vi "get controller information.vi"(6 "Network Adapters (F)":bool caption="network adapters (F)", 8 "error in":errorcluster, 11 "controller in":refnum<class "Controller.lvclass">) -> (0 "error out":errorcluster, 2 "controller information":T1={"system session"=refnum, "system hardware ref"=refnum, "vendor name"="", "product name"="", "product ID"=0, "serial number"="", "device information"={"resource"="", "device class"="", "system start time"=timestamp(0 s since 1904-01-01), "current time"=timestamp(0 s since 1904-01-01), "time zone"="", "firmware revision"="", "image title"="", "image version"="", "system status"=""}, "primary network adapter"={"IP address"="", "MAC address"="", "IP address request mode"=1, "subnet mask"="", "gateway"="", "DNS server"="", "adapter mode"=1, "adapter type"=1}, "secondary network adapters"=[]} {"product ID" format="%.0x"; "primary network adapter"."IP address request mode" items=["Static"=1, "DHCP/Link Local"=2, "Link-Local Only"=4, "DHCP Only"=8]; "primary network adapter"."adapter type" items=["Ethernet"=1, "WLAN"=2]; "primary network adapter"."adapter mode" items=["Disabled"=1, "TCP/IP Ethernet"=2, "Deterministic"=4, "EtherCAT"=8, "TCP/IP WLAN Connect"=32, "TCP/IP WLAN Create"=64]; "secondary network adapters"."IP address request mode" items=["Static"=1, "DHCP/Link Local"=2, "Link-Local Only"=4, "DHCP Only"=8]; "secondary network adapters"."adapter type" items=["Disabled"=1, "TCP/IP Ethernet"=2, "Deterministic"=4, "EtherCAT"=8, "TCP/IP WLAN Connect"=32, "TCP/IP WLAN Create"=64]; "secondary network adapters"."adapter mode" items=["Disabled"=1, "TCP/IP Ethernet"=2, "Deterministic"=4, "EtherCAT"=8, "TCP/IP WLAN Connect"=32, "TCP/IP WLAN Create"=64]}, 3 "controller out":refnum<class "Controller.lvclass">)   [LabVIEW 2013, in "SMI.lvlib" / "Controller.lvclass"]
uses:
  Controller.lvclass
  controller information.ctl
  device information.ctl
  network adapter settings.ctl
  Controller.lvclass/Controller.ctl
  SysCfg Device/read system session.vi
  Device/read vendor name.vi
  Device/read product name.vi
  Device/read product ID.vi
  Device/read serial number.vi
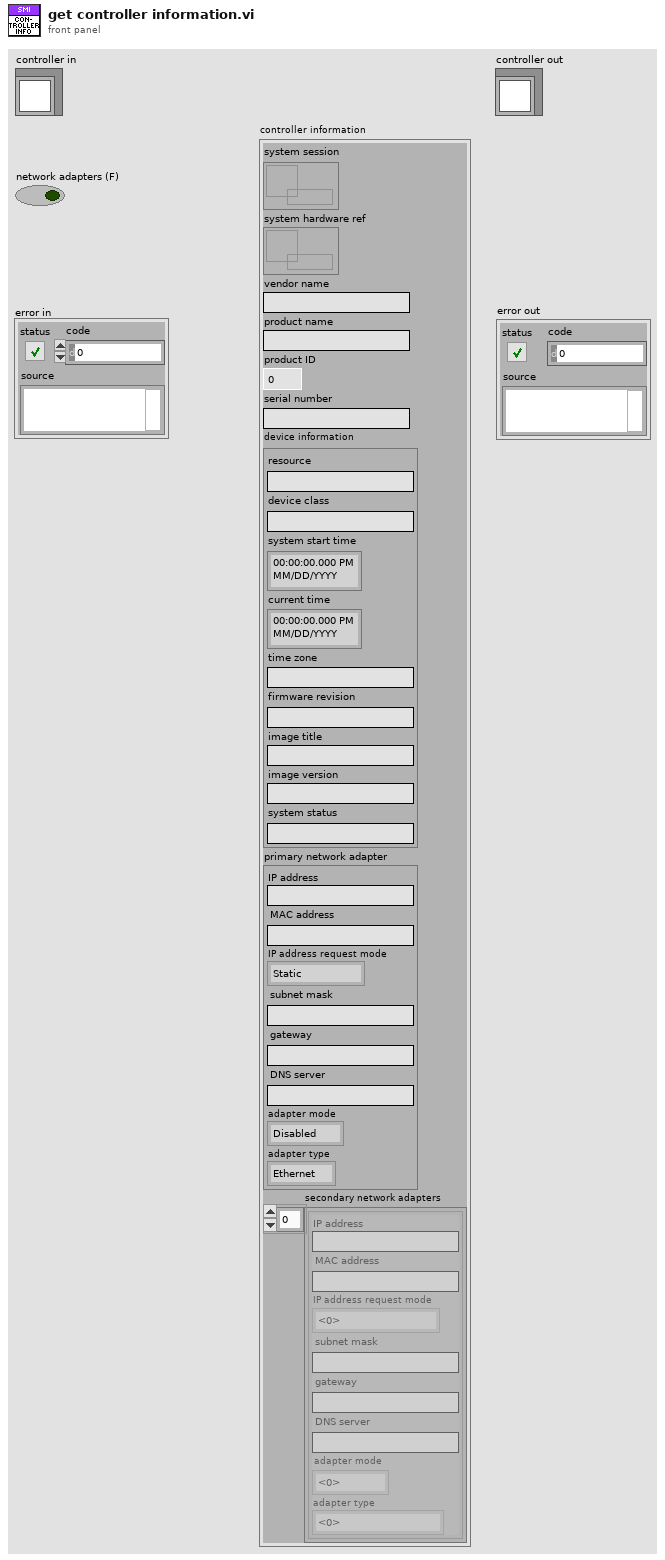
[diagram p1: front panel]
types:
  T1 = typedef "SMI.lvlib/Controller.lvclass/controller information.ctl" = cluster{"system session":refnum<data-value>, "system hardware ref":refnum<data-value>, "vendor name":string, "product name":string, "product ID":u16, "serial number":string, "device information":T2, "primary network adapter":T3, "secondary network adapters":T3[]}
  T2 = typedef "SMI.lvlib/Controller.lvclass/device information.ctl" = cluster{"resource":string, "device class":string, "system start time":timestamp, "current time":timestamp, "time zone":string, "firmware revision":string, "image title":string, "image version":string, "system status":string}
  T3 = typedef "SMI.lvlib/Controller.lvclass/network adapter settings.ctl" = cluster{"IP address":string, "MAC address":string, "IP address request mode":u32, "subnet mask":string, "gateway":string, "DNS server":string, "adapter mode":u32, "adapter type":u32}
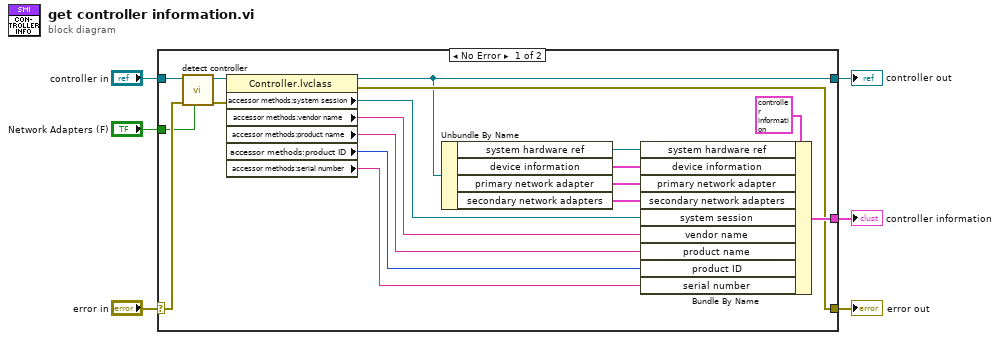
[diagram p0: block diagram]
diagram:
  n1 = case shown="No Error" "error in" {
    selector: "error in" -> [w11 w26]
    tunnel: [w24 _] -> w6
    tunnel: [w23 w26] -> w5
    tunnel: "controller in" -> [w8 w25]
    tunnel: [w13 w25] -> w4
    tunnel: "Network Adapters (F)" -> [w7 _]
    frame No Error {
      n2 = call "detect controller.vi"("Network Adapters"=w7, "error in"=w11, "controller in"=w8) -> ("error out"=w10:errorcluster, "controller out"=w9:refnum<class "Controller.lvclass">)  [unwired: 7 in]
      n3 = property class="Controller.lvclass"(reference=w9, error in=w10) -> (reference out=w13:refnum<class "Controller.lvclass">, error out=w23:errorcluster, "accessor methods:system session"=w12:refnum<data-value>, "accessor methods:vendor name"=w19:string, "accessor methods:product name"=w22:string, "accessor methods:product ID"=w21:u16, "accessor methods:serial number"=w20:string)
      n4 = Unbundle By Name(w13) -> ("system hardware ref"=w15:refnum<data-value>, "device information"=w18:T2, "primary network adapter"=w17:T3, "secondary network adapters"=w16:T3[])
      n5 = Bundle By Name(cluster=T1 {"system session"=refnum, "system hardware ref"=refnum, "vendor name"="", "product name"="", "product ID"=0, "serial number"="", "device information"={"resource"="", "device class"="", "system start time"=timestamp(0 s since 1904-01-01), "current time"=timestamp(0 s since 1904-01-01), "time zone"="", "firmware revision"="", "image title"="", "image version"="", "system status"=""}, "primary network adapter"={"IP address"="", "MAC address"="", "IP address request mode"=1, "subnet mask"="", "gateway"="", "DNS server"="", "adapter mode"=1, "adapter type"=1}, "secondary network adapters"=[]} ("Device Information"), "system hardware ref"=w15, "device information"=w18, "primary network adapter"=w17, "secondary network adapters"=w16, "system session"=w12, "vendor name"=w19, "product name"=w22, "product ID"=w21, "serial number"=w20) -> (w24:T1)
    }
    frame Error {
    }
  }
  "error out" <- w5
  "controller out" <- w4
  "controller information" <- w6
